vi "Kinesis - MPZ601 MNA601 - Two Axis Scan.vi"() -> ()   [LabVIEW 2012]
doc: "2D piezo scan example Vi to find a signal."
uses:
  U:/Kinesis LabVIEW Website Examples/Thorlabs.MotionControl.Controls.dll
  Thorlabs.MotionControl.Controls.dll
  U:/Kinesis LabVIEW Website Examples/Thorlabs.MotionControl.ModularRackCLI.dll
  Thorlabs.MotionControl.ModularRackCLI.dll
  U:/Kinesis LabVIEW Website Examples/Thorlabs.MotionControl.GenericNanoTrakCLI.dll
  Thorlabs.MotionControl.GenericNanoTrakCLI.dll
panel:
  in  "SelectedRange":i32(ring)=10 items=["TIA_Range1_3NA"=3, "TIA_Range2_10NA"=4, "TIA_Range3_30NA"=5, "TIA_Range4_100NA"=6, "TIA_Range5_300NA"=7, "TIA_Range6_1MUA"=8, "TIA_Range7_3MUA"=9, "TIA_Range8_10MUA"=10, "TIA_Range9_30MUA"=11, "TIA_Range10_100MUA"=12, "TIA_Range11_300MUA"=13, "TIA_Range12_1MA"=14, "TIA_Range13_3MA"=15, "TIA_Range14_10MA"=16]
  in  "Number Of Steps":i32=50
  in  "Scale":sgl=0.25 format="%.2f"
  in  "ModularPiezoControl Ch.1":refnum<k24>(container)
  in  "ModularPiezoControl Ch.2":refnum<k24>(container)
  in  "ModularNanoTrakControl":refnum<k24>(container)
  out "Error":errorcluster
  in  "MPZ601 Serial Number":string
  in  "MNA601 Serial Number":string
  # "Thorlabs Hardware: \nMPZ601 Rack Module 2-Ch Piezoelectric Controller With Feedback\nhttps://www.thorlabs.com/newgrouppage9.cfm?objectgroup_id=1185\n\nMNA601 Rack Module Fiber Auto-alignment Module\nhttps://www.thorlabs.com/newgrouppage9.cfm?objectgroup_id=1187\n\nDescription: The below VI will enable you to connect to a MNA601 & MPZ601. This VI will initiate a simple 2D raster scan of the MPZ601 piezo outputs. An example of this application setup is pictured whereby the MPZ601 will drive the internal X & Z piezo blocks of a MAX302 stage. The MAX302 stage is holding an optical fibre aligned to a waveguide in series with secondary receiving fibre via use of Thorlabs flexure stage holder accessories. The secondary fibre is mounted to a secondary co-located MAX302 stage. This fibre is connected to the Optical Input of the MNA601 controller.\n\nThe piezo output raster scan will stop either when the max number of steps have been reached or the user selected TIA Range of the MNA601 has been reached, indicating that the MNA601 is reading sufficient photocurrent from the fibre-copupling system. This signifies an \"optimised throughput\" in the system. The MNA601 is defaulted to 'Latch' mode as the MNA601 HV Outputs are not in use.\n\nInstructions: \n1) Connect a MNA601 & MPZ601 to MMR601 as per the respective product user manuals. These can be connected to any bay in the MMR601 rack.\n2) Enter the module serial numbers below.\n3) Enter the Scan parameters, as well as the exitting TIA Range.\n4) To run the VI, click the run button in the LabVIEW Toolbar.\n5) The VI will exit when either the required TIA Range has been reached or the scan has completed."
  # "Notes:"
  # "- Ensure that the appropriate .DLLs are copied into your Project Folder. Check that the correct bit type are used depending on your version of LabVIEW\ni.e. 32-bit or 64-bit.\n\n\n\n\n\n\n\n\n\n\n\n\n\n\n- Open the example VI through the LabVIEW Project Explorer to correctly load the User Interface from Thorlabs.MotionControl.Controls.dll."
  # "Example Image of .NET Controller - VI opened via Project Explorer/ not opened via Project Explorer"
  # "VI Not Opened via Project Explorer"
  # "VI Opened via Project Explorer"
  # "- To explore the range of methods available, please visit the .NET API, included with your Kinesis software.\n\n- For tips on building your own VIs with Thorlabs Motion Control Hardware, please see our LabVIEW Guide here.\nhttps://www.thorlabs.com/newgrouppage9.cfm?objectgroup_id=10285"
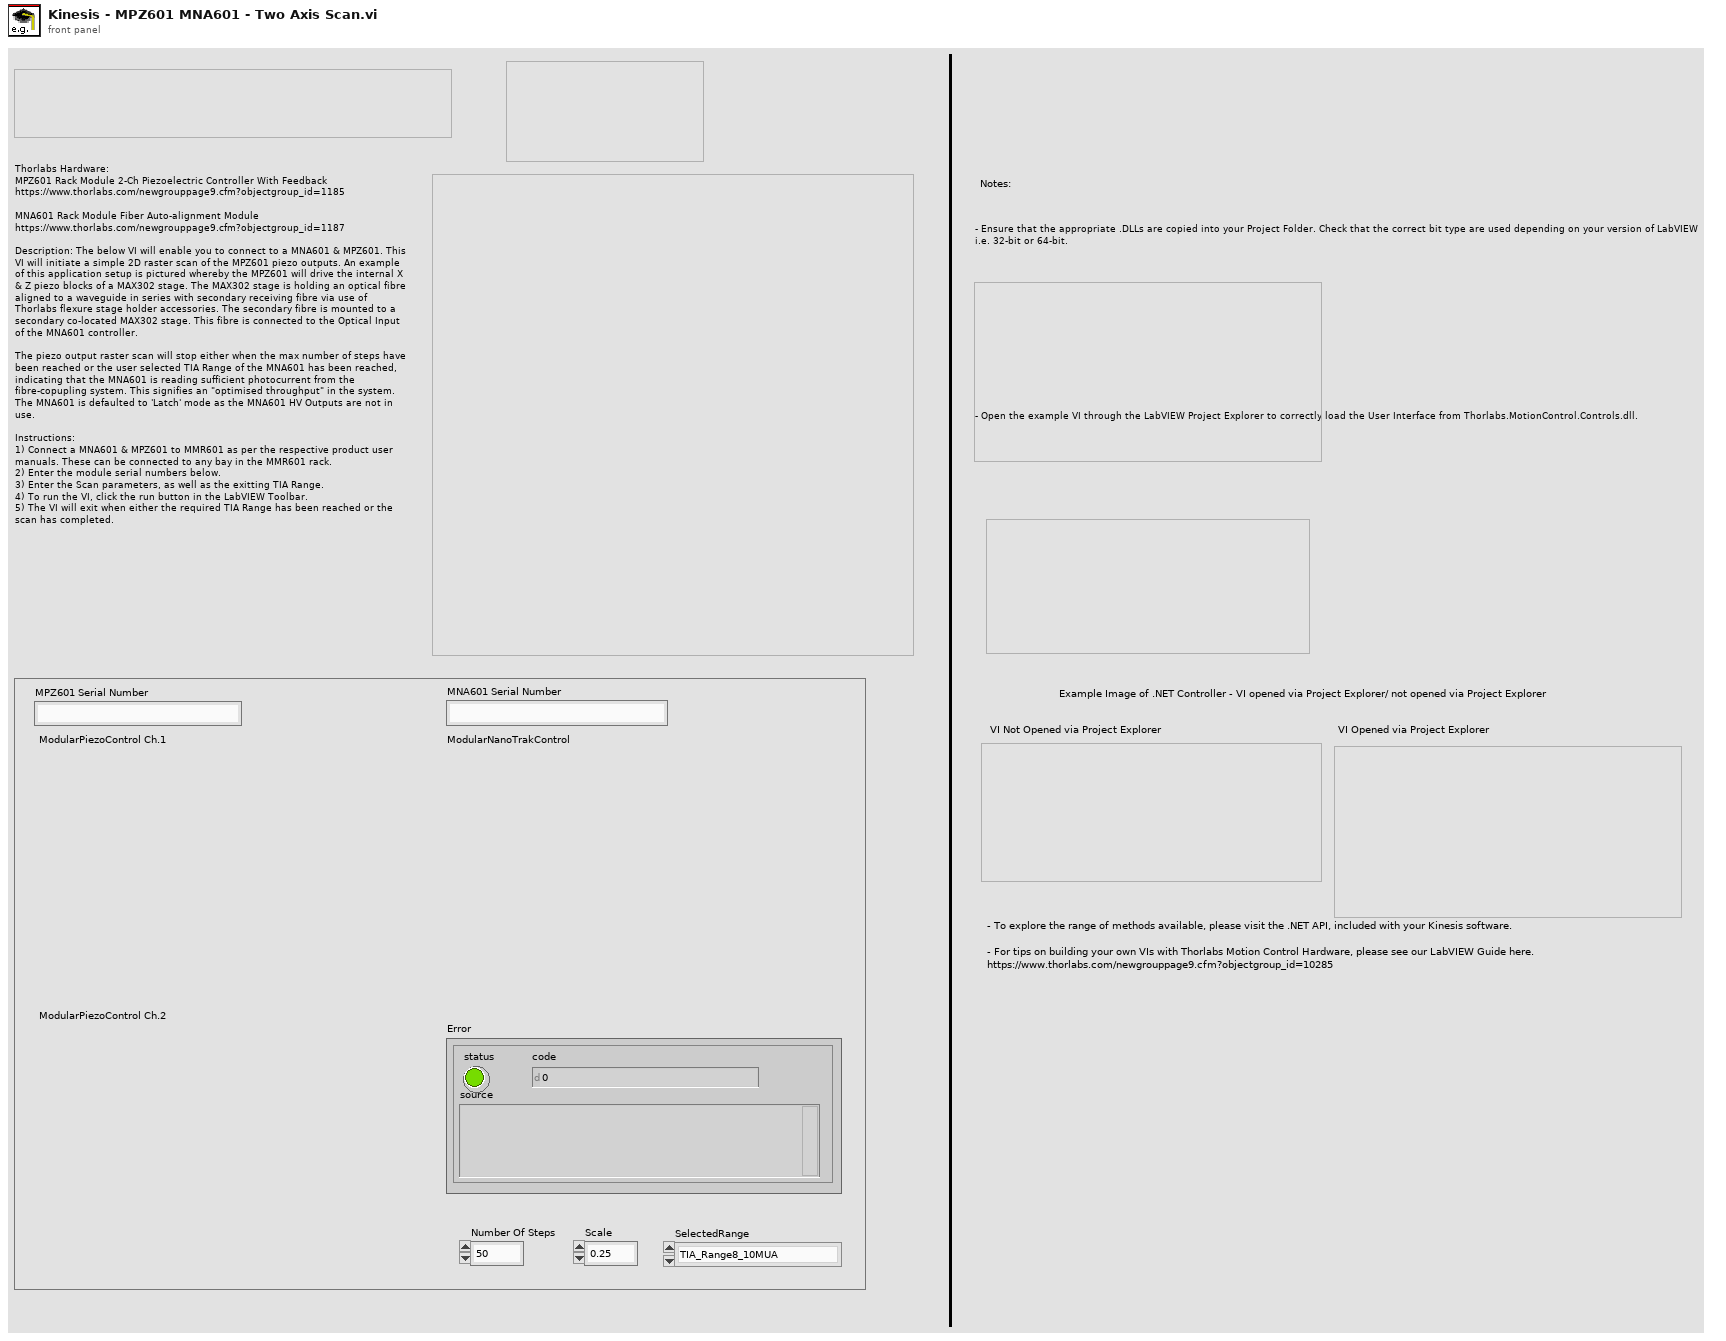
[diagram p1: front panel]
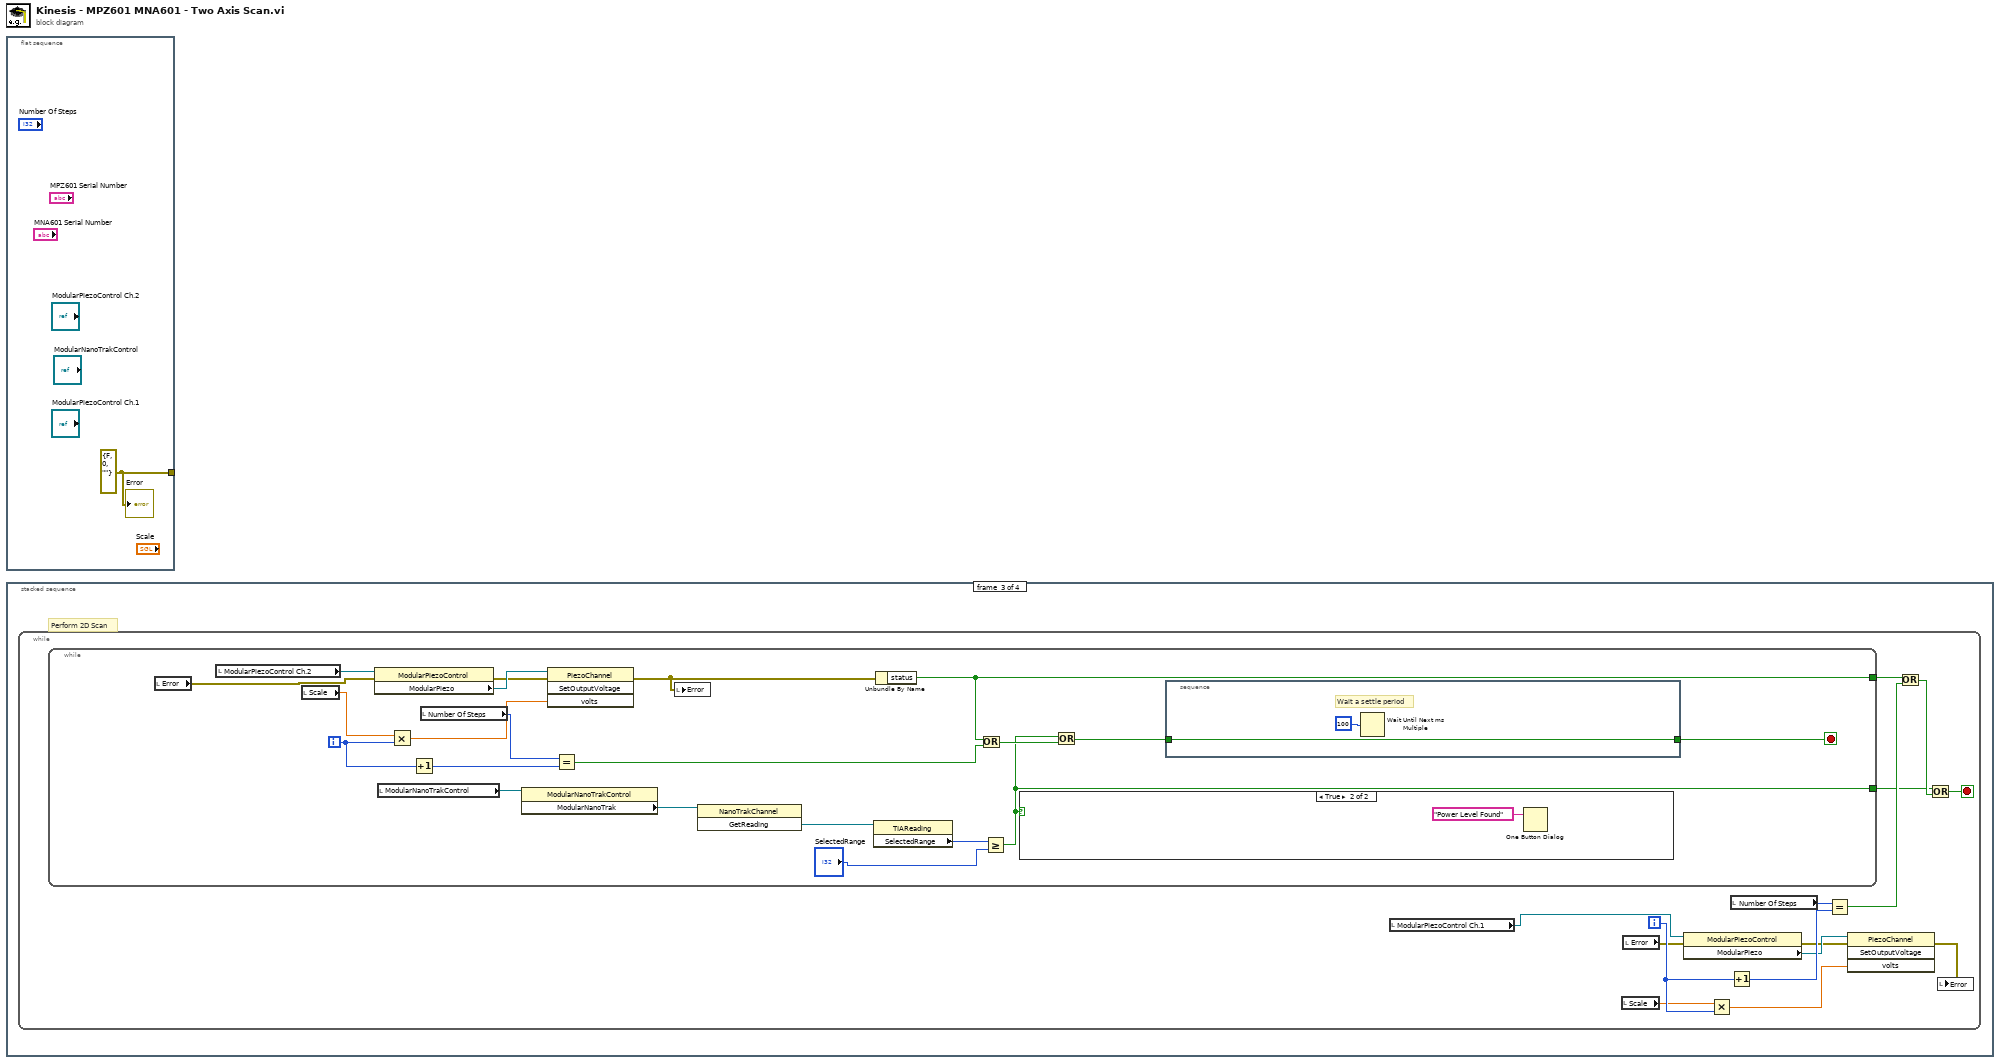
[diagram p0: block diagram]
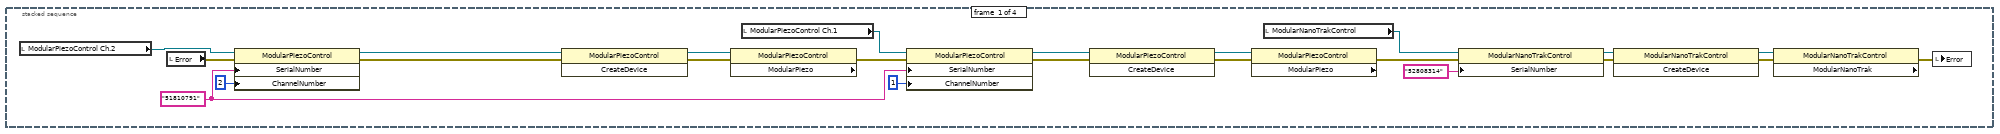
[diagram p2: hidden frame]
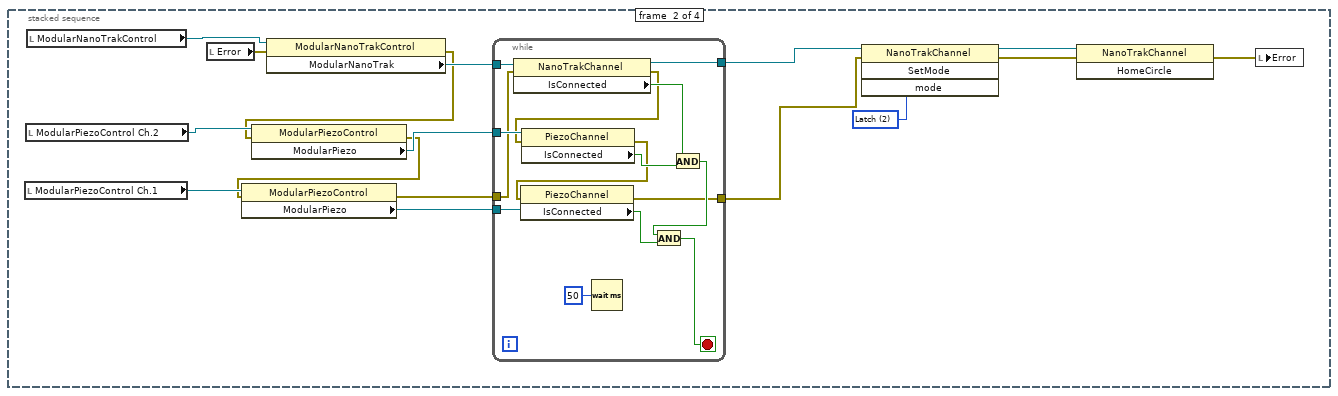
[diagram p3: hidden frame]
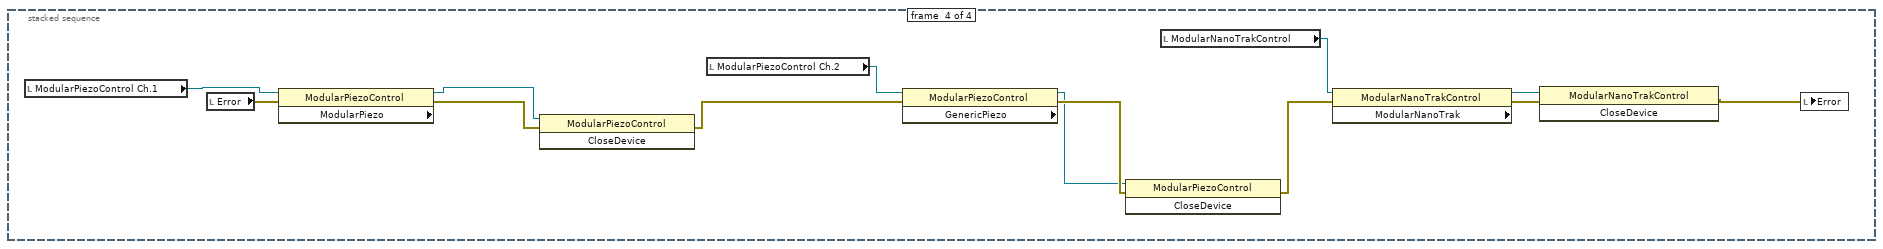
[diagram p5: hidden frame]
diagram:
  n1 = flat-sequence {
    tunnel: [w1] -> _
    frame #0 {
      w1 = errorcluster {"status"=FALSE, "code"=0, "source"=""} ("error in (no error)")
      "Error" <- w1
    }
  }
  n2 = stacked-sequence {
    frame #0 {
      w3 = "51810791" ("SerialNumber")
      n3 = local read "ModularPiezoControl Ch.2"() -> (w5:refnum<k24>)
      n4 = local read "Error"() -> (w19:errorcluster)
      n5 = property class="ModularPiezoControl"(reference=w5, error in=w19, "SerialNumber"=w3, "ChannelNumber"=2) -> (reference out=w24:refnum<k24>, error out=w23:errorcluster)
      n6 = invoke class="ModularPiezoControl" method="CreateDevice"(reference=w24, error in=w23) -> (reference out=w21:refnum<k24>, error out=w22:errorcluster)  [unwired: 1 in, 1 out]
      n7 = property class="ModularPiezoControl" props=["ModularPiezo"](reference=w21, error in=w22) -> (error out=w15:errorcluster)  [unwired: 2 out]
      n8 = local read "ModularPiezoControl Ch.1"() -> (w4:refnum<k24>)
      n9 = property class="ModularPiezoControl"(reference=w4, error in=w15, "SerialNumber"=w3, "ChannelNumber"=1) -> (reference out=w8:refnum<k24>, error out=w18:errorcluster)
      n10 = invoke class="ModularPiezoControl" method="CreateDevice"(reference=w8, error in=w18) -> (reference out=w7:refnum<k24>, error out=w17:errorcluster)  [unwired: 1 in, 1 out]
      n11 = property class="ModularPiezoControl" props=["ModularPiezo"](reference=w7, error in=w17) -> (error out=w6:errorcluster)  [unwired: 2 out]
      n12 = local read "ModularNanoTrakControl"() -> (w14:refnum<k24>)
      n13 = property class="ModularNanoTrakControl"(reference=w14, error in=w6, "SerialNumber"="52808314") -> (reference out=w13:refnum<k24>, error out=w11:errorcluster)
      n14 = invoke class="ModularNanoTrakControl" method="CreateDevice"(reference=w13, error in=w11) -> (reference out=w12:refnum<k24>, error out=w10:errorcluster)  [unwired: 1 in, 1 out]
      n15 = property class="ModularNanoTrakControl" props=["ModularNanoTrak"](reference=w12, error in=w10) -> (error out=w9:errorcluster)  [unwired: 2 out]
      n16 = local write "Error"(w9) -> ()
    }
    frame #1 {
      w35 = 2 items=["Undefined", "Piezo", "Latch", "Tracking", "HorizontalTracking", "VerticalTracking"] ("mode")
      n17 = local read "ModularPiezoControl Ch.1"() -> (w33:refnum<k24>)
      n18 = local read "ModularPiezoControl Ch.2"() -> (w34:refnum<k24>)
      n19 = local read "ModularNanoTrakControl"() -> (w40:refnum<k24>)
      n20 = local read "Error"() -> (w38:errorcluster)
      n21 = property class="ModularNanoTrakControl"(reference=w40, error in=w38) -> (error out=w27:errorcluster, "ModularNanoTrak"=w32:refnum<k24>)  [unwired: 1 out]
      n22 = property class="ModularPiezoControl"(reference=w34, error in=w27) -> (error out=w26:errorcluster, "ModularPiezo"=w31:refnum<k24>)  [unwired: 1 out]
      n23 = property class="ModularPiezoControl"(reference=w33, error in=w26) -> (error out=w25:errorcluster, "ModularPiezo"=w30:refnum<k24>)  [unwired: 1 out]
      n24 = while {
        tunnel: w32 -> [w54]
        tunnel: w31 -> [w53]
        tunnel: w30 -> [w52]
        tunnel: [w45] -> w29
        tunnel: [w43] -> w28
        tunnel: w25 -> [w41]
        stop <- w47 stop-if-true
        n25 = property class="NanoTrakChannel"(reference=w54, error in=w41) -> (reference out=w45:refnum<k24>, error out=w42:errorcluster, "IsConnected"=w51:bool)
        n26 = property class="PiezoChannel"(reference=w53, error in=w42) -> (error out=w44:errorcluster, "IsConnected"=w50:bool)  [unwired: 1 out]
        n27 = property class="PiezoChannel"(reference=w52, error in=w44) -> (error out=w43:errorcluster, "IsConnected"=w48:bool)  [unwired: 1 out]
        n28 = Wait (ms)(milliseconds to wait=u32 50) -> ()  [unwired: 1 out]
        n29 = And(x=w51, y=w50) -> (x .and. y?=w49:bool)
        n30 = And(x=w49, y=w48) -> (x .and. y?=w47:bool)
      }
      n31 = invoke class="NanoTrakChannel" method="SetMode"(reference=w29, error in=w28, "mode"=w35) -> (reference out=w39:refnum<k24>, error out=w37:errorcluster)  [unwired: 1 in, 2 out]
      n32 = invoke class="NanoTrakChannel" method="HomeCircle"(reference=w39, error in=w37) -> (error out=w36:errorcluster)  [unwired: 1 in, 2 out]
      n33 = local write "Error"(w36) -> ()
    }
    frame #2 {
      # "Perform 2D Scan"
      n34 = while {
        i -> [w66]
        stop <- w65 stop-if-true
        n35 = while {
          tunnel: [w85] -> w63
          tunnel: [w89] -> w69
          i -> [w88]
          stop <- w83 stop-if-true
          n36 = local read "Error"() -> (w70:errorcluster)
          n37 = local read "ModularPiezoControl Ch.2"() -> (w74:refnum<k24>)
          n38 = local read "Scale"() -> (w73:sgl)
          n39 = property class="ModularPiezoControl"(reference=w74, error in=w70) -> (error out=w81:errorcluster, "ModularPiezo"=w82:refnum<k24>)  [unwired: 1 out]
          n40 = local read "ModularNanoTrakControl"() -> (w79:refnum<k24>)
          n41 = Multiply(x=w73, y=w88) -> (x*y=w80:sgl)
          n42 = Increment(x=w88) -> (x+1=w87:i32)
          n43 = local read "Number Of Steps"() -> (w75:i32)
          n44 = property class="ModularNanoTrakControl"(reference=w79) -> ("ModularNanoTrak"=w78:refnum<k24>)  [unwired: 1 in, 2 out]
          n45 = invoke class="PiezoChannel" method="SetOutputVoltage"(reference=w82, error in=w81, "volts"=w80) -> (error out=w76:errorcluster)  [unwired: 1 in, 3 out]
          n46 = Equal?(x=w75, y=w87) -> (x = y?=w90:bool)
          n47 = local write "Error"(w76) -> ()
          n48 = invoke class="NanoTrakChannel" method="GetReading"(reference=w78) -> ("GetReading"=w77:refnum<k24>)  [unwired: 2 in, 2 out]
          n49 = property class="TIAReading"(reference=w77) -> ("SelectedRange"=w71:i32)  [unwired: 1 in, 2 out]
          n50 = Unbundle By Name(w76) -> ("status"=w89:bool)
          n51 = Or(x=w89, y=w90) -> (x .or. y?=w86:bool)
          n52 = Greater Or Equal?(x=w71, y="SelectedRange") -> (x >= y?=w85:bool)
          n53 = case shown="True" w85 {
            frame False {
            }
            frame True {
              n54 = One Button Dialog(message="Power Level Found") -> ()  [unwired: 1 in, 1 out]
            }
          }
          n55 = Or(x=w85, y=w86) -> (x .or. y?=w84:bool)
          n56 = stacked-sequence {
            tunnel: w84 -> [w91]
            tunnel: [w91] -> w83
            frame #0 {
              # "Wait a settle period"
              n57 = Wait Until Next ms Multiple(millisecond multiple=u32 100) -> ()  [unwired: 1 out]
            }
          }
        }
        n58 = local read "ModularPiezoControl Ch.1"() -> (w61:refnum<k24>)
        n59 = local read "Scale"() -> (w56:sgl)
        n60 = local read "Error"() -> (w59:errorcluster)
        n61 = property class="ModularPiezoControl"(reference=w61, error in=w59) -> (error out=w58:errorcluster, "ModularPiezo"=w60:refnum<k24>)  [unwired: 1 out]
        n62 = Multiply(x=w56, y=w66) -> (x*y=w62:sgl)
        n63 = Increment(x=w66) -> (x+1=w67:i32)
        n64 = local read "Number Of Steps"() -> (w57:i32)
        n65 = Equal?(x=w57, y=w67) -> (x = y?=w68:bool)
        n66 = invoke class="PiezoChannel" method="SetOutputVoltage"(reference=w60, error in=w58, "volts"=w62) -> (error out=w55:errorcluster)  [unwired: 1 in, 3 out]
        n67 = Or(x=w69, y=w68) -> (x .or. y?=w64:bool)
        n68 = Or(x=w63, y=w64) -> (x .or. y?=w65:bool)
        n69 = local write "Error"(w55) -> ()
      }
    }
    frame #3 {
      n70 = local read "ModularPiezoControl Ch.1"() -> (w104:refnum<k24>)
      n71 = local read "Error"() -> (w103:errorcluster)
      n72 = property class="ModularPiezoControl" props=["ModularPiezo"](reference=w104, error in=w103) -> (reference out=w96:refnum<k24>, error out=w95:errorcluster)  [unwired: 1 out]
      n73 = invoke class="ModularPiezoControl" method="CloseDevice"(reference=w96, error in=w95) -> (error out=w94:errorcluster)  [unwired: 1 in, 2 out]
      n74 = local read "ModularPiezoControl Ch.2"() -> (w105:refnum<k24>)
      n75 = property class="ModularPiezoControl" props=["GenericPiezo"](reference=w105, error in=w94) -> (reference out=w100:refnum<k24>, error out=w102:errorcluster)  [unwired: 1 out]
      n76 = invoke class="ModularPiezoControl" method="CloseDevice"(reference=w100, error in=w102) -> (error out=w101:errorcluster)  [unwired: 1 in, 2 out]
      n77 = local read "ModularNanoTrakControl"() -> (w106:refnum<k24>)
      n78 = property class="ModularNanoTrakControl" props=["ModularNanoTrak"](reference=w106, error in=w101) -> (reference out=w98:refnum<k24>, error out=w99:errorcluster)  [unwired: 1 out]
      n79 = invoke class="ModularNanoTrakControl" method="CloseDevice"(reference=w98, error in=w99) -> (error out=w97:errorcluster)  [unwired: 1 in, 2 out]
      n80 = local write "Error"(w97) -> ()
    }
  }
